vi "Register Backlog.vi"(7 "TimingEngine":T1, 8 "error in (no error)":errorcluster, 9 "DAQ Diag":T2, 10 "Task Name":string, 11 "Cfg Grandmaster in":refnum<class "Cfg Grandmaster.lvclass">) -> (0 "error out":errorcluster, 3 "Cfg Grandmaster out":refnum<class "Cfg Grandmaster.lvclass">)   [LabVIEW 2012, in "Configuration Grandmaster.lvlib" / "Cfg Grandmaster.lvclass"]
uses:
  Cfg Grandmaster.lvclass
  Common/Controls/DAQ Diagnostics.ctl
  Common/Controls/TE_Designator.ctl
  Cfg Grandmaster.lvclass/Cfg Grandmaster.ctl
  Class FP Ctrls/FP Controls.lvclass
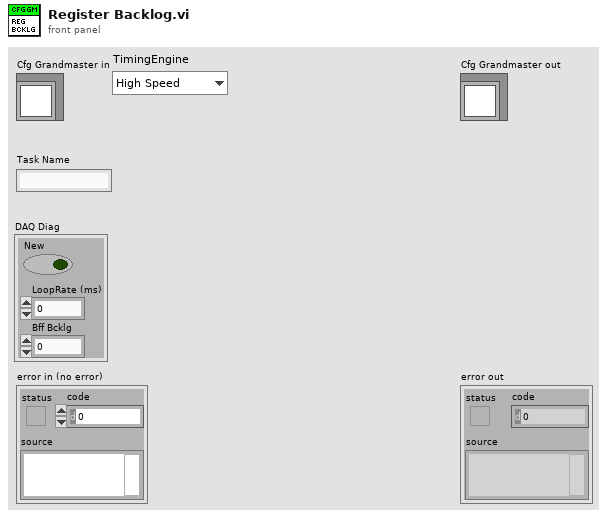
[diagram p1: front panel]
types:
  T1 = typedef "TE_Designator.ctl" = enum16{"High Speed", "Low Speed"}
  T2 = typedef "DAQ Diagnostics.ctl" = cluster{"New":bool, "LoopRate (ms)":u32, "Bff Bcklg":dbl}
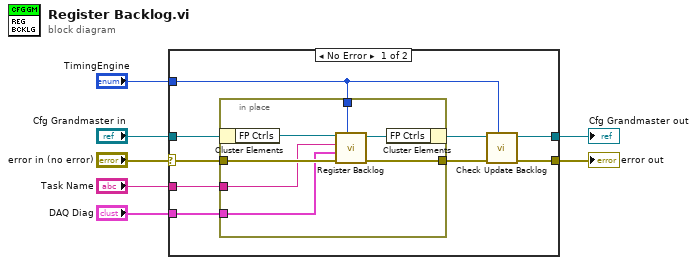
[diagram p0: block diagram]
diagram:
  n1 = case shown="No Error" "error in (no error)" {
    selector: "error in (no error)" -> [w13 w25]
    tunnel: [w15 w25] -> w6
    tunnel: [w16 w24] -> w4
    tunnel: "Cfg Grandmaster in" -> [w11 w24]
    tunnel: "DAQ Diag" -> [w8 _]
    tunnel: "Task Name" -> [w9 _]
    tunnel: "TimingEngine" -> [w14 _]
    frame No Error {
      n2 = in-place {
        in-place-border: w14 -> [w23]
        in-place-border: w13 -> [w22]
        in-place-border: [w21] -> w12
        in-place-border: w9 -> [w18]
        in-place-border: w8 -> [w17]
        n3 = in-place-cluster #1(w11) -> ("FP Ctrls"=w20:refnum<class "FP Controls.lvclass">)
        n4 = call "Register Backlog.vi"("TimingEngine"=w23, "error in (no error)"=w22, "DAQ Diag"=w17, "Task Name"=w18, "FP Controls in"=w20) -> ("error out"=w21:errorcluster, "FP Controls out"=w19:refnum<class "FP Controls.lvclass">)  [unwired: 5 in]
        n5 = in-place-cluster #1("FP Ctrls"=w19) -> (w10:refnum<class "Cfg Grandmaster.lvclass">)
      }
      n6 = call "Check Update Backlog.vi"("TimingEngine"=w14, "error in (no error)"=w12, "Cfg Grandmaster in"=w10) -> ("error out"=w15:errorcluster, "Cfg Grandmaster out"=w16:refnum<class "Cfg Grandmaster.lvclass">)  [unwired: 7 in]
    }
    frame Error {
    }
  }
  "error out" <- w6
  "Cfg Grandmaster out" <- w4
